vi "FF_Moiz.vi"(11 "file path (use dialog)":T2=path "C:/JK/circle.txt") -> (0 "xyz_o":dbl[][](array[numeric]), 3 "Array":T1[](array[typedef]))   [LabVIEW 2013]
uses:
  typeDef/AnkleTraj.ctl
  Moiz/Control 1.ctl
  <vilib>/Analysis/baseanly.llb/Real Dot Product.vi
  <vilib>/Utility/file.llb/Read From Spreadsheet File (DBL).vi
  <vilib>/Analysis/NI_AALBase.lvlib
panel:
  out "Array 2":T1[](array[typedef])
  out "deleted portion":dbl[](array[numeric])
  out "initialized array":dbl[](array[numeric])
  out "pos":dbl[][](array[numeric])
  out "deleted portion 2":dbl[](array[numeric])
  out "all rows":dbl[][](array[numeric]) format="%0.3f"
  out "x_o":dbl[](array[numeric])
  out "array w/ subset deleted":dbl[][](array[numeric])
  in  "AnkleTraj":T1
  # "JIyeon->po.txt   V->poV3.txt"
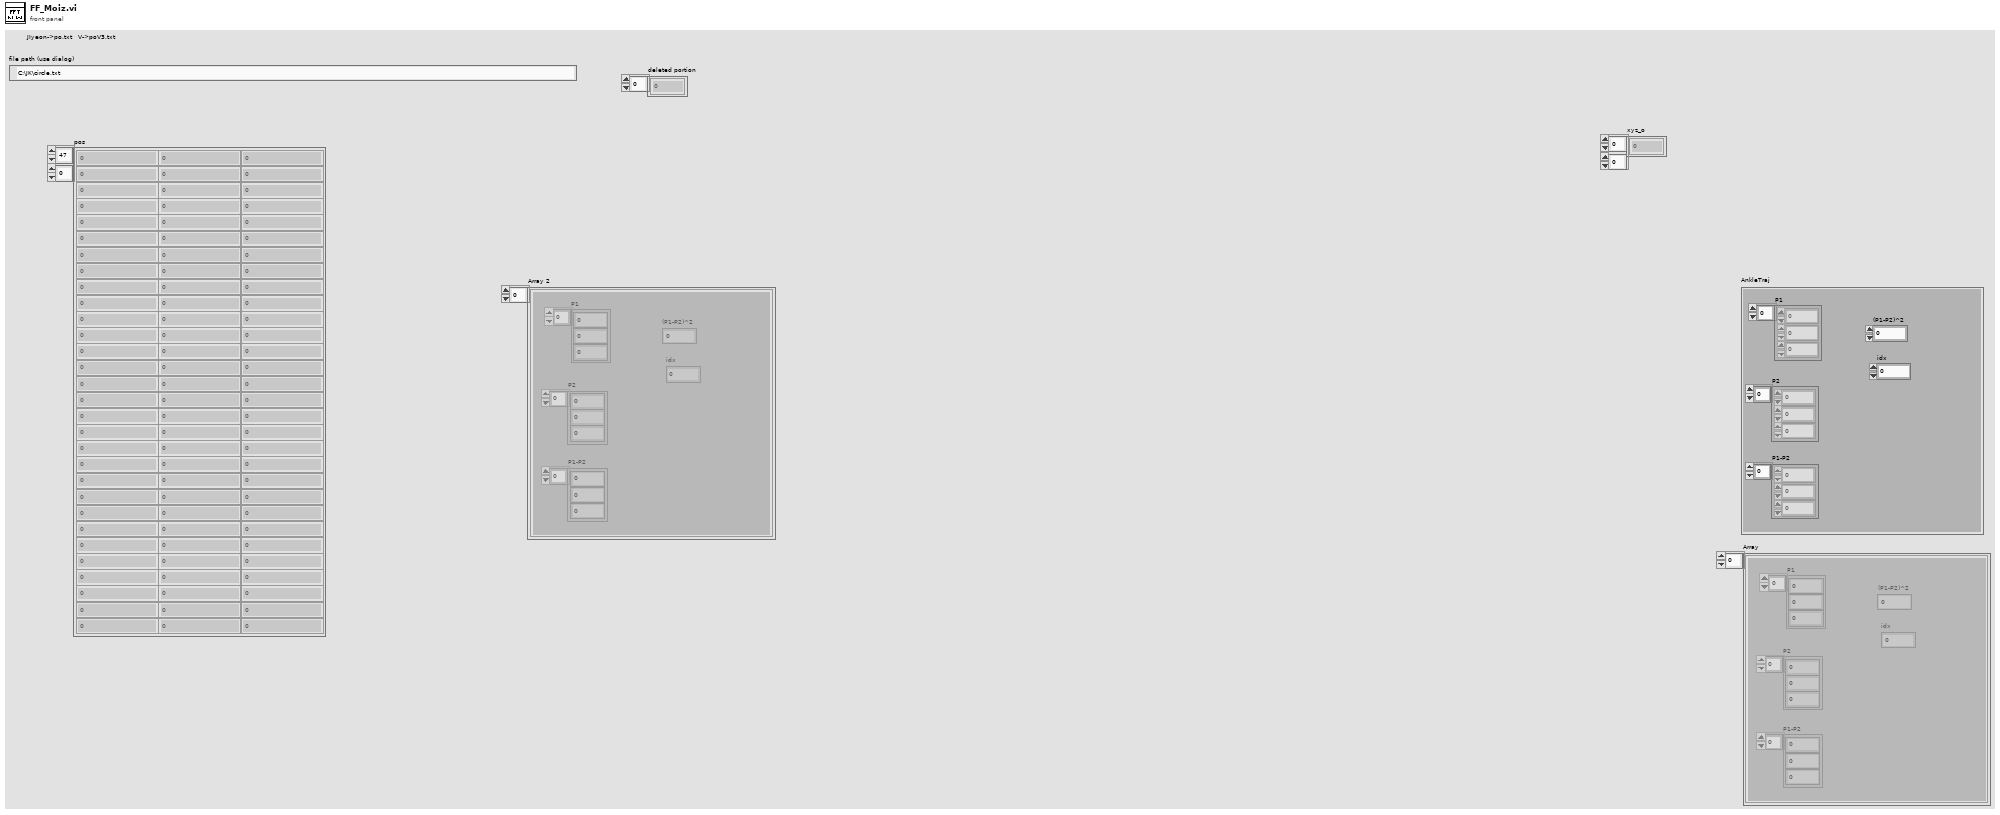
[diagram p1: front panel]
types:
  T1 = typedef "AnkleTraj.ctl" = cluster{"P1":dbl[], "P2":dbl[], "P1-P2":dbl[], "(P1-P2)^2":dbl, "idx":i32}
  T2 = typedef "Control 1.ctl" = path
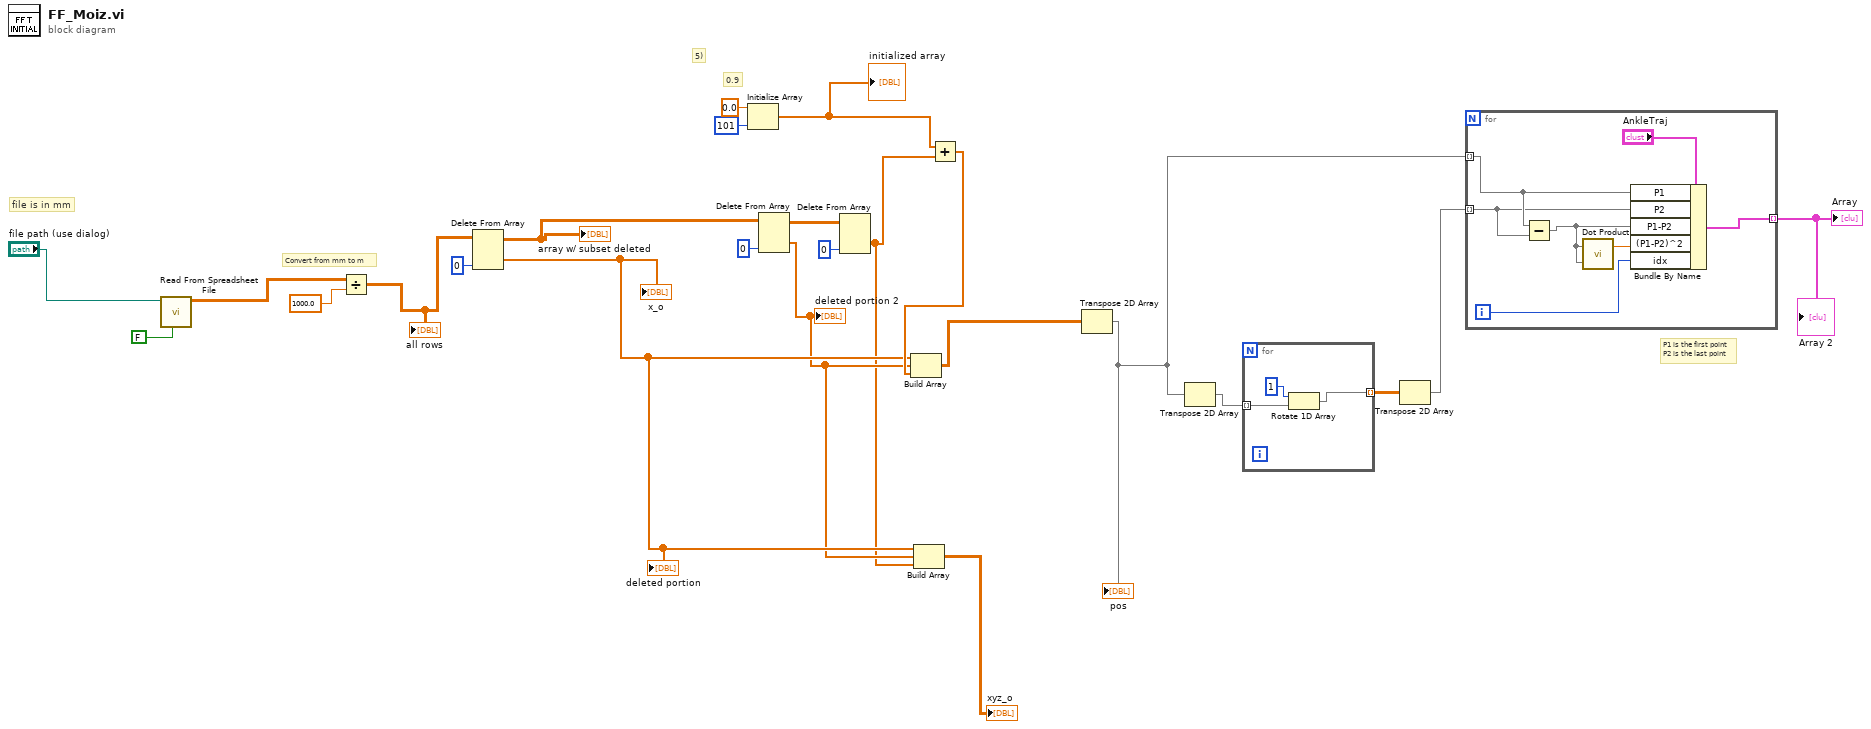
[diagram p0: block diagram]
diagram:
  # "P1 is the first point\nP2 is the last point"
  # "Convert from mm to m"
  # "5)"
  # "0.9"
  # "file is in mm"
  n1 = call-poly <vilib>:"Read From Spreadsheet File.vi"("transpose (no:F)"=FALSE, "file path (dialog if empty)"="file path (use dialog)") -> ("all rows"=w2:dbl[][])  [unwired: 5 in, 4 out]
  n2 = Divide(x=w2, y=1000.0) -> (x/y=w1:dbl[][])
  "all rows" <- w1
  n3 = Delete From Array(array=w1, index (col)=0 ("disabled index (col)")) -> (deleted portion=w7:dbl[], array with subset deleted=w18:dbl[][])  [unwired: 2 in]
  "array w/ subset deleted" <- w18
  "x_o" <- w7
  "deleted portion" <- w7
  n4 = Initialize Array(0.0 ("element"), 101 ("dimension size")) -> (w9:dbl[])
  "initialized array" <- w9
  n5 = Delete From Array(array=w18, index (col)=0) -> (deleted portion=w6:dbl[], array with subset deleted=w17:dbl[][])  [unwired: 2 in]
  "deleted portion 2" <- w6
  n6 = Delete From Array(array=w17, index (col)=0 ("disabled index (col)")) -> (deleted portion=w5:dbl[])  [unwired: 2 in, 1 out]
  n7 = Build Array(w7, w6, w5) -> (→"xyz_o":dbl[][])
  n8 = Add(x=w9, y=w5) -> (x+y=w8:dbl[])
  n9 = Build Array(w7, w6, w8) -> (w12:dbl[][])
  n10 = Transpose 2D Array(2D array=w12) -> (transposed array=w13:dbl[][])
  "pos" <- w13
  n11 = Transpose 2D Array(2D array=w13) -> (transposed array=w24:dbl[][])
  n12 = for {
    tunnel: w24 -> [w27] mode=indexing
    tunnel: [w26] -> w23 mode=indexing
    n13 = Rotate 1D Array(1:w27, 2:1 ("n")) -> (0:w26:dbl[])
  }
  n14 = Transpose 2D Array(2D array=w23) -> (transposed array=w22:dbl[][])
  n15 = for {
    tunnel: w13 -> [w33] mode=indexing
    tunnel: w22 -> [w32] mode=indexing
    tunnel: [w29] -> w21 mode=indexing
    i -> [w28]
    n16 = Subtract(x=w33, y=w32) -> (x-y=w30:dbl[])
    n17 = call-poly <vilib>:"Dot Product.vi"("Y Vector"=w30, "X Vector"=w30) -> ("X * Y"=w31:dbl)  [unwired: 1 out]
    n18 = Bundle By Name(cluster="AnkleTraj", "P1"=w33, "P2"=w32, "P1-P2"=w30, "(P1-P2)^2"=w31, "idx"=w28) -> (w29:T1)
  }
  "Array" <- w21
  "Array 2" <- w21
